vi "dcy04.vi"() -> ()   [LabVIEW 2023]
uses:
  parametertype.ctl
  Public/SECoP-data/SECoP-data.ctl
  <vilib>/regexp/Match Regular Expression.xnode
  SECoP.lvlib
panel:
  out "log":string
  in  "DLL path":path=path "D:/shall-repos/shall-labview/64bit"
  in  "stop":bool
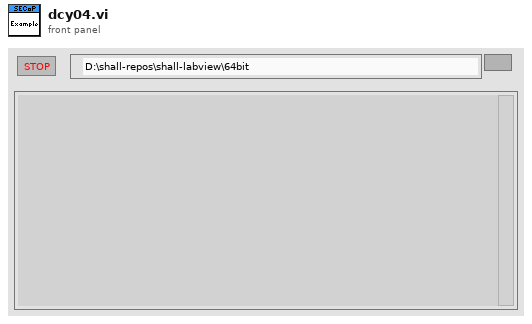
[diagram p1: front panel]
types:
  T1 = typedef "parametertype.ctl" = enum8{"readonly", "readwrite", "command"}
  T2 = typedef "SECoP.lvlib/SECoP-data.ctl" = cluster{"ptr32":u32, "ptr64":u64}
  T3 = cluster{"name":string, "type":T1, "datatype":string, "description":string, "SECoP_dataPtr":T2}[]
  T4 = typedef "SECoP.lvlib/SECoP-libraries.ctl" = cluster{"serverDLL":path, "variantDLL":path, "cleanup_mode":bool, "Context_ID":string}
  T5 = cluster{"name":string, "type":T1, "datatype":string, "description":string, "SECoP_dataPtr":T2}
  T6 = typedef "SECoP.lvlib/SECoP-action.ctl" = enum32{"any action", "read", "change", "do cmd"}
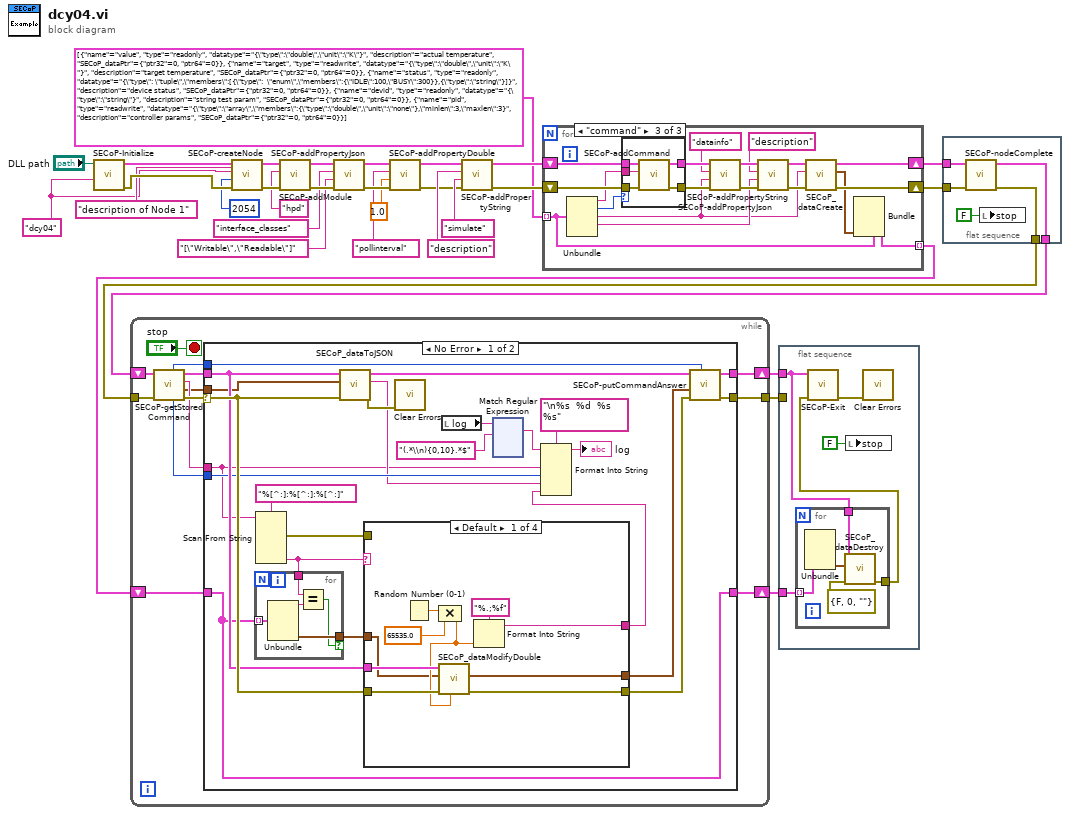
[diagram p0: block diagram]
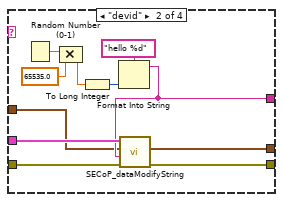
[diagram p2: hidden frame]
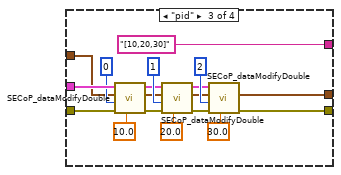
[diagram p3: hidden frame]
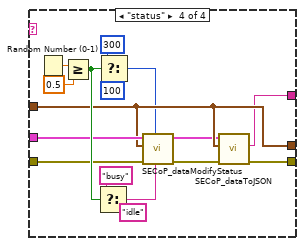
[diagram p4: hidden frame]
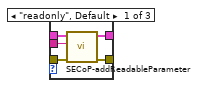
[diagram p6: hidden frame]
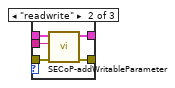
[diagram p7: hidden frame]
diagram:
  w1 = "dcy04"
  n1 = call "SECoP-Initialize.vi"("Context ID (in)"=w1, "DLL path (in)"="DLL path") -> ("error out"=w30:errorcluster, "DLL path (out)"=w31:T4)  [unwired: 8 in]
  n2 = call "SECoP-createNode.vi"("description"="description of Node 1", "error in (no error)"=w30, "TCP port"=u16 2054, "node id"=w1, "DLL path (in)"=w31) -> ("error out"=w26:errorcluster, "DLL path (out)"=w29:T4)  [unwired: 5 in]
  n3 = call "SECoP-addModule.vi"("error in (no error)"=w26, "module name"="hpd" ("name"), "DLL path (in)"=w29) -> ("error out"=w23:errorcluster, "DLL path (out)"=w24:T4)  [unwired: 7 in]
  n4 = call "SECoP-addPropertyJson.vi"("error in (no error)"=w23, "property value"="[\"Writable\",\"Readable\"]" ("name"), "property name"="interface_classes" ("name"), "DLL path (in)"=w24) -> ("error out"=w12:errorcluster, "DLL path (out)"=w14:T4)  [unwired: 6 in]
  n5 = call "SECoP-addPropertyDouble.vi"("error in (no error)"=w12, "property value"=1.0, "property name"="pollinterval", "DLL path (in)"=w14) -> ("error out"=w11:errorcluster, "DLL path (out)"=w13:T4)  [unwired: 6 in]
  n6 = call "SECoP-addPropertyString.vi"("error in (no error)"=w11, "property value"="simulate" ("name"), "property name"="description" ("name"), "DLL path (in)"=w13) -> ("error out"=w17:errorcluster, "DLL path (out)"=w18:T4)  [unwired: 6 in]
  n7 = for {
    tunnel: T3 [{"name"="value", "type"=enum."readonly", "datatype"="{\"type\":\"double\",\"unit\":\"K\"}", "description"="actual temperature", "SECoP_dataPtr"={"ptr32"=0, "ptr64"=0}}, {"name"="target", "type"=enum."readwrite", "datatype"="{\"type\":\"double\",\"unit\":\"K\"}", "description"="target temperature", "SECoP_dataPtr"={"ptr32"=0, "ptr64"=0}}, {"name"="status", "type"=enum."readonly", "datatype"="{\"type\": \"tuple\",\"members\":[{\"type\":  \"enum\",\"members\":{\"IDLE\":100,\"BUSY\":300}},{\"type\":\"string\"}]}", "description"="device status", "SECoP_dataPtr"={"ptr32"=0, "ptr64"=0}}, {"name"="devid", "type"=enum."readonly", "datatype"="{\"type\":\"string\"}", "description"="string test param", "SECoP_dataPtr"={"ptr32"=0, "ptr64"=0}}, {"name"="pid", "type"=enum."readwrite", "datatype"="{\"type\":\"array\",\"members\":{\"type\":\"double\",\"unit\":\"none\"},\"minlen\":3,\"maxlen\":3}", "description"="controller params", "SECoP_dataPtr"={"ptr32"=0, "ptr64"=0}}] -> [w36] mode=indexing
    shift-right: [w33] -> w6
    shift-left: w18 -> [w48]
    shift-right: [w38] -> w5
    shift-left: w17 -> [w47]
    tunnel: [w34] -> w4 mode=indexing
    n8 = Unbundle(w36) -> ("name"=w37:string, "type"=w49:T1, "datatype"=w39:string, "description"=w42:string)  [unwired: 1 out]
    n9 = case shown="\"command\"" w49 {
      tunnel: w37 -> [w54 w61 w66]
      tunnel: w48 -> [w56 w60 w65]
      tunnel: [w55 w59 w64] -> w46
      tunnel: [w52 w57 w62] -> w45
      tunnel: w47 -> [w53 w58 w63]
      frame "readonly", Default {
        n10 = call "SECoP-addReadableParameter.vi"("error in (no error)"=w53, "parameter name"=w54, "DLL path (in)"=w56) -> ("error out"=w52:errorcluster, "DLL path (out)"=w55:T4)  [unwired: 7 in]
      }
      frame "readwrite" {
        n11 = call "SECoP-addWritableParameter.vi"("error in (no error)"=w58, "parameter name"=w61, "DLL path (in)"=w60) -> ("error out"=w57:errorcluster, "DLL path (out)"=w59:T4)  [unwired: 7 in]
      }
      frame "command" {
        n12 = call "SECoP-addCommand.vi"("error in (no error)"=w63, "command name"=w66, "DLL path (in)"=w65) -> ("error out"=w62:errorcluster, "DLL path (out)"=w64:T4)  [unwired: 7 in]
      }
    }
    n13 = call "SECoP-addPropertyJson.vi"("error in (no error)"=w45, "property value"=w39, "property name"="datainfo" ("name"), "DLL path (in)"=w46) -> ("error out"=w50:errorcluster, "DLL path (out)"=w51:T4)  [unwired: 6 in]
    n14 = call "SECoP-addPropertyString.vi"("error in (no error)"=w50, "property value"=w42, "property name"="description" ("name"), "DLL path (in)"=w51) -> ("error out"=w41:errorcluster, "DLL path (out)"=w40:T4)  [unwired: 6 in]
    n15 = call "SECoP_dataCreate.vi"("error in (no error)"=w41, "Description"=w39, "DLL path (in)"=w40) -> ("error out"=w38:errorcluster, "SECoP_dataPtr (out)"=w35:T2, "DLL path (out)"=w33:T4)  [unwired: 6 in]
    n16 = Bundle(cluster=w36, "SECoP_dataPtr"=w35) -> (w34:T5)  [unwired: 4 in]
  }
  n17 = while {
    shift-right: [w79] -> w20
    shift-left: w7 -> [w77]
    tunnel: w8 -> [w76]
    tunnel: [w69] -> w19
    shift-right: [w67] -> w3
    shift-left: w4 -> [w68]
    stop <- "stop" stop-if-true
    n18 = call "SECoP-getStoredCommand.vi"("error in (no error)"=w76, "DLL path (in)"=w77) -> ("error out"=w74:errorcluster, "SECoP_data"=w70:T2, "command/parameter path"=w71:string, "DLL path (out)"=w75:T4, "action"=w72:T6, "command id"=w73:u64)  [unwired: 4 in]
    n19 = case shown="No Error" w74 {
      selector: w74 -> [w103 w277]
      tunnel: w75 -> [w102 w278]
      tunnel: [w97 w278] -> w79
      tunnel: w73 -> [w96 _]
      tunnel: w71 -> [w85 _]
      tunnel: w70 -> [w82 _]
      tunnel: w72 -> [w95 _]
      tunnel: [w100 w277] -> w69
      tunnel: w68 -> [w81 w276]
      tunnel: [w81 w276] -> w67
      frame No Error {
        n20 = Scan From String(format string="%[^:]:%[^:]:%[^:]", input string=w85) -> (error out=w89:errorcluster, output 3=w84:string)  [unwired: 7 in, 2 out]
        n21 = for {
          tunnel: w81 -> [w104] mode=indexing
          tunnel: w84 -> [w107]
          tunnel: [w106] -> w83 if=w105
          n22 = Unbundle(w104) -> ("name"=w108:string, "SECoP_dataPtr"=w106:T2)  [unwired: 3 out]
          n23 = Equal?(x=w107, y=w108) -> (x = y?=w105:bool)
        }
        n24 = call "SECoP_dataToJSON.vi"("error in (no error)"=w103, "SECoP_dataPtr"=w82, "DLL path (in)"=w102) -> ("error out"=w101:errorcluster, "JSONBuffer"=w86:string, "DLL path (out)"=w87:T4)  [unwired: 6 in]
        n25 = case shown="Default" w84 {
          tunnel: [w114 w120 "[10,20,30]" w145] -> w80
          tunnel: w89 -> [_ _ _ _]
          tunnel: w102 -> [w113 w122 w142 w150]
          tunnel: [w109 w118 w128 w148] -> w98
          tunnel: w103 -> [w112 w121 w140 w149]
          tunnel: [w111 w119 w129 w151] -> w99
          tunnel: w83 -> [w109 w118 w128 w148]
          frame Default {
            n26 = Random Number (0-1)() -> (number: 0 to 1=w116:dbl)
            n27 = Compound Arithmetic op=MULTIPLY(w116, 65535.0 ("value")) -> (w110:dbl)
            n28 = call "SECoP_dataModifyDouble.vi"("Value"=w110, "error in (no error)"=w112, "SECoP_data"=w109, "DLL path (in)"=w113) -> ("error out"=w111:errorcluster)  [unwired: 6 in, 1 out]
            n29 = Format Into String(format string="%.;%f", w110) -> (resulting string=w114:string)  [unwired: 2 in, 1 out]
          }
          frame "devid" {
            n30 = Random Number (0-1)() -> (number: 0 to 1=w124:dbl)
            n31 = Compound Arithmetic op=MULTIPLY(w124, 65535.0 ("value")) -> (w126:dbl)
            n32 = To Long Integer(number=w126) -> (32bit integer=w127:i32)
            n33 = Format Into String(format string="hello %d", w127) -> (resulting string=w120:string)  [unwired: 2 in, 1 out]
            n34 = call "SECoP_dataModifyString.vi"("error in (no error)"=w121, "Value"=w120, "SECoP_dataPtr"=w118, "DLL path (in)"=w122) -> ("error out"=w119:errorcluster)  [unwired: 6 in, 1 out]
          }
          frame "pid" {
            n35 = call "SECoP_dataModifyDouble.vi"("Value"=10.0, "error in (no error)"=w140, "Index"=u32 0, "SECoP_data"=w128, "DLL path (in)"=w142) -> ("error out"=w131:errorcluster, "DLL path (out)"=w133:T4)  [unwired: 5 in]
            n36 = call "SECoP_dataModifyDouble.vi"("Value"=20.0, "error in (no error)"=w131, "Index"=u32 1, "SECoP_data"=w128, "DLL path (in)"=w133) -> ("error out"=w130:errorcluster, "DLL path (out)"=w132:T4)  [unwired: 5 in]
            n37 = call "SECoP_dataModifyDouble.vi"("Value"=30.0, "error in (no error)"=w130, "Index"=u32 2, "SECoP_data"=w128, "DLL path (in)"=w132) -> ("error out"=w129:errorcluster)  [unwired: 5 in, 1 out]
          }
          frame "status" {
            n38 = Random Number (0-1)() -> (number: 0 to 1=w158:dbl)
            n39 = Greater Or Equal?(x=w158, y=0.5) -> (x >= y?=w154:bool)
            n40 = Select(t="busy", s=w154, f="idle") -> (s? t:f=w144:string)
            n41 = Select(t=i64 300 ("Value"), s=w154, f=i64 100 ("Value")) -> (s? t:f=w143:i64)
            n42 = call "SECoP_dataModifyStatus.vi"("status text"=w144, "status code"=w143, "error in (no error)"=w149, "SECoP_dataPtr (in)"=w148, "DLL path (in)"=w150) -> ("error out"=w146:errorcluster, "DLL path (out)"=w147:T4)  [unwired: 4 in, 1 out]
            n43 = call "SECoP_dataToJSON.vi"("error in (no error)"=w146, "SECoP_dataPtr"=w148, "DLL path (in)"=w147) -> ("error out"=w151:errorcluster, "JSONBuffer"=w145:string)  [unwired: 6 in, 1 out]
          }
        }
        n44 = call <vilib>:"Clear Errors.vi"("error in (no error)"=w101) -> ()  [unwired: 5 in, 2 out]
        n45 = local read "log"() -> (w92:string)
        n46 = xnode "Match Regular Expression"("input string"=w92, "regular expression"="(.*\\n){0,10}.*$") -> ("whole match"=w93:string)  [unwired: 4 in, 4 out]
        n47 = Format Into String(format string="\n%s  %d  %s  %s", initial string=w93, w85, w95, w86, w80) -> (resulting string=→"log":string)  [unwired: 1 in, 1 out]
        n48 = call "SECoP-putCommandAnswer.vi"("command id"=w96, "error in (no error)"=w99, "value (SECoP_data)"=w98, "DLL path (in)"=w87) -> ("error out"=w100:errorcluster, "DLL path (out)"=w97:T4)  [unwired: 6 in]
      }
      frame Error {
      }
    }
  }
  n49 = flat-sequence {
    tunnel: w20 -> [w280]
    tunnel: w19 -> [_]
    tunnel: w3 -> [w282]
    frame #0 {
      n50 = for {
        tunnel: w282 -> [w288] mode=indexing
        tunnel: [w286] -> w281
        tunnel: w280 -> [w285]
        n51 = Unbundle(w288) -> ("SECoP_dataPtr"=w287:T2)  [unwired: 4 out]
        n52 = call "SECoP_dataDestroy.vi"("error in (no error)"=errorcluster {"status"=FALSE, "code"=0, "source"=""}, "SECoP_dataPtr"=w287, "DLL path (in)"=w285) -> ("error out"=w286:errorcluster)  [unwired: 7 in, 1 out]
      }
      n53 = call "SECoP-Exit.vi"("error in (no error)"=w281, "DLL path (in)"=w280) -> ("error out"=w279:errorcluster)  [unwired: 9 in]
      n54 = local write "stop"(FALSE) -> ()
      n55 = call <vilib>:"Clear Errors.vi"("error in (no error)"=w279) -> ()  [unwired: 5 in, 2 out]
    }
  }
  n56 = flat-sequence {
    tunnel: w6 -> [w292]
    tunnel: w5 -> [w291]
    tunnel: [w289] -> w7
    tunnel: [w290] -> w8
    frame #0 {
      n57 = call "SECoP-nodeComplete.vi"("error in (no error)"=w291, "DLL path (in)"=w292) -> ("error out"=w290:errorcluster, "DLL path (out)"=w289:T4)  [unwired: 8 in]
      n58 = local write "stop"(FALSE) -> ()
    }
  }
